vi "Write growables.vi"(5 "growables":refnum<class "GrowableFunction.lvclass">[](array[class]), 9 "Diagram in":refnum<class "Diagram.lvclass">) -> (3 "Diagram out":refnum<class "Diagram.lvclass">)   [LabVIEW 2014, in "Diagram.lvclass"]
uses:
  Diagram.lvclass
  GrowableFunction/GrowableFunction.lvclass
  Diagram.lvclass/Diagram.ctl
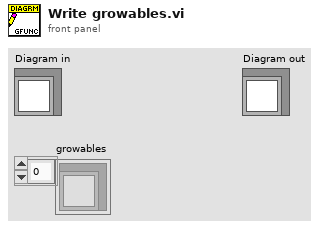
[diagram p1: front panel]
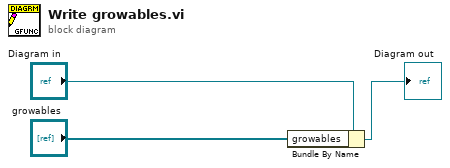
[diagram p0: block diagram]
diagram:
  n1 = Bundle By Name(cluster="Diagram in", "growables"="growables") -> (→"Diagram out":refnum<class "Diagram.lvclass">)
